vi "Multi-line.vi"(0 "String":string) -> (1 "Array":string[](array[string]), 2 "Array size":i32)   [LabVIEW 2012]
panel:
  out "DummyArray":string[](array[string])
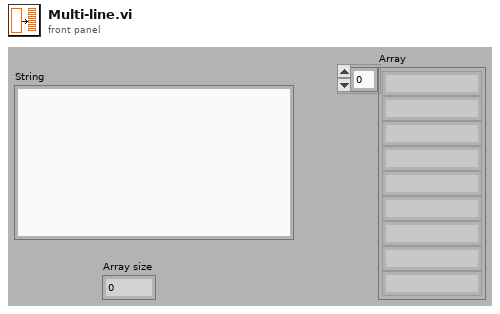
[diagram p1: front panel]
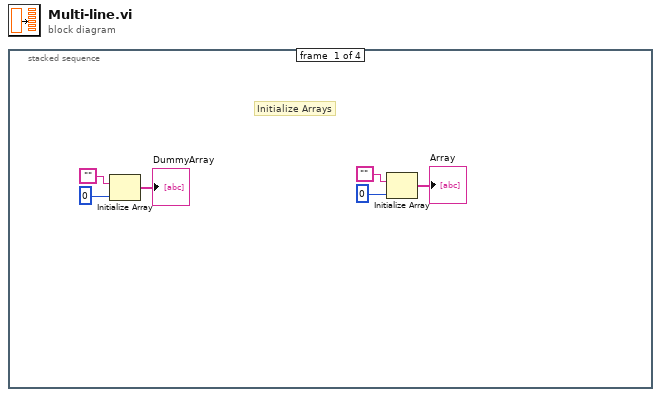
[diagram p0: block diagram]
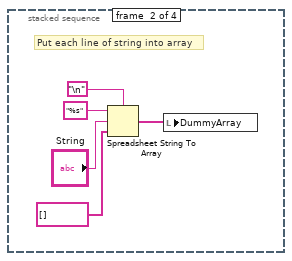
[diagram p2: hidden frame]
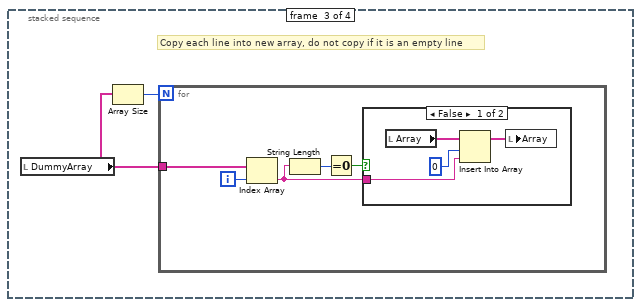
[diagram p3: hidden frame]
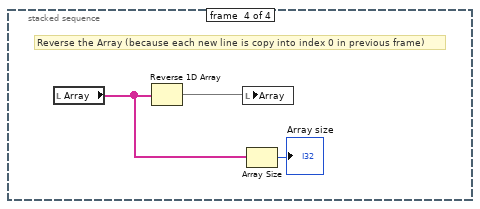
[diagram p5: hidden frame]
diagram:
  n1 = stacked-sequence {
    frame #0 {
      # "Initialize Arrays"
      n2 = Initialize Array("", 0 ("dimension size")) -> (→"DummyArray":string[])
      n3 = Initialize Array("", 0 ("dimension size")) -> (→"Array":string[])
    }
    frame #1 {
      # "Put each line of string into array"
      n4 = Spreadsheet String To Array(delimiter (Tab)="\n", format string="%s", spreadsheet string="String", array type (2D Dbl)=string[] [] ("Array")) -> (array=w7:string[])
      n5 = local write "DummyArray"(w7) -> ()
    }
    frame #2 {
      # "Copy each line into new array, do not copy if it is an empty line"
      n6 = local read "DummyArray"() -> (w12:string[])
      n7 = Array Size(array=w12) -> (size(s)=w13:i32)
      n8 = for {
        N: w13 -> [_]
        tunnel: w12 -> [w17]
        i -> [w16]
        n9 = Index Array(array=w17, index=w16) -> (element=w14:string)
        n10 = String Length(string=w14) -> (length=w18:i32)
        n11 = Equal To 0?(x=w18) -> (x = 0?=w15:bool)
        n12 = case shown="False" w15 {
          tunnel: w14 -> [w22 _]
          frame False {
            n13 = local read "Array"() -> (w21:string[])
            n14 = Insert Into Array(array=w21, index=0, new element=w22) -> (w20:string[])
            n15 = local write "Array"(w20) -> ()
          }
          frame True {
          }
        }
      }
    }
    frame #3 {
      # "Reverse the Array (because each new line is copy into index 0 in previous frame)"
      n16 = local read "Array"() -> (w24:string[])
      n17 = Reverse 1D Array(array=w24) -> (reversed array=w25:string[])
      n18 = local write "Array"(w25) -> ()
      n19 = Array Size(array=w24) -> (size(s)=→"Array size":i32)
    }
  }
